vi "Remove DC Component.vi"(8 "error in":errorcluster, 10 "InverterWaveforms":T1) -> (0 "error out":errorcluster, 2 "InverterWaveforms out":T1)   [LabVIEW 2019, in "Main.lvclass"]
doc: "Developed by Kevin Thompson\nkevin@thompsonengineering.net\n\nCopyright 2020\nThompson Engineering, LLC"
uses:
  Main.lvclass
  Common/DataTypes/InverterWaveforms--cluster.ctl
  Common/DataTypes/ChannelWaveforms--cluster.ctl
  <vilib>/Analysis/NI_AALPro.lvlib
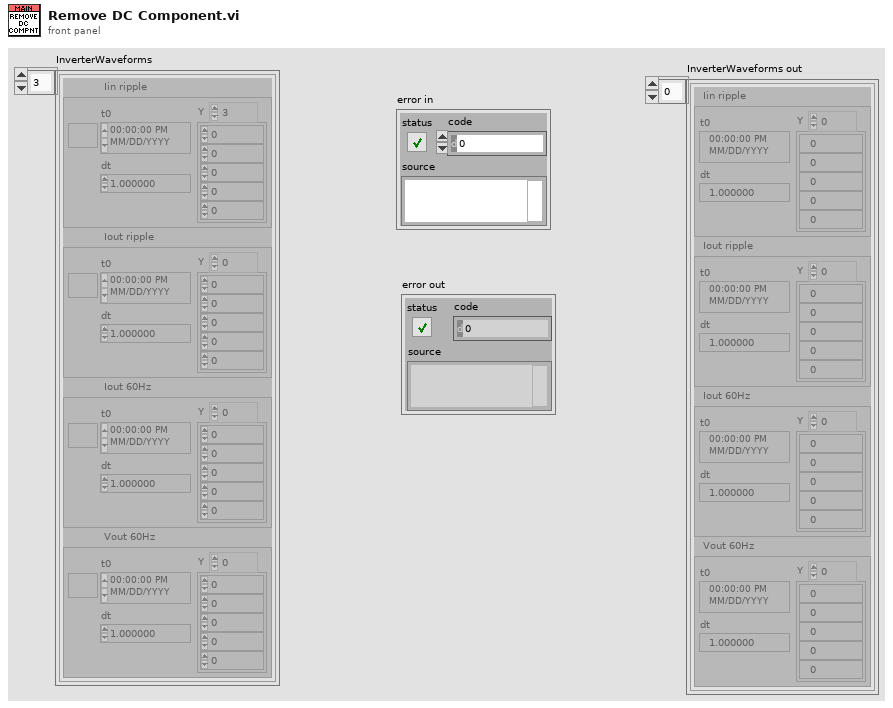
[diagram p1: front panel]
types:
  T1 = typedef "InverterWaveforms--cluster.ctl" = T2[]
  T2 = typedef "ChannelWaveforms--cluster.ctl" = cluster{"Iin ripple ":waveform(dbl), "Iout ripple ":waveform(dbl), "Iout 60Hz":waveform(dbl), "Vout 60Hz":waveform(dbl)}
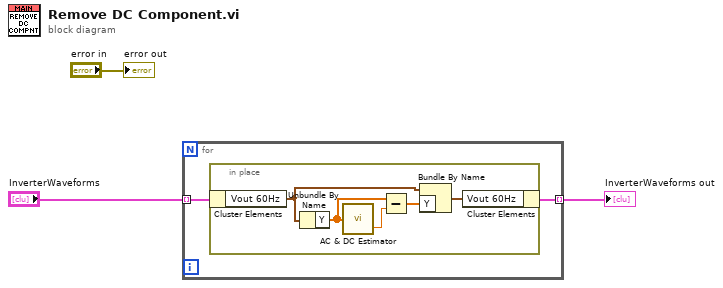
[diagram p0: block diagram]
diagram:
  n1 = for {
    tunnel: "InverterWaveforms" -> [w5] mode=indexing
    tunnel: [w4] -> w1 mode=indexing
    n2 = in-place {
      n3 = in-place-cluster #1(w5) -> ("Vout 60Hz"=w8:waveform(dbl))
      n4 = Unbundle By Name(w8) -> ("Y"=w9:dbl[])
      n5 = call <vilib>:"AC & DC Estimator.vi"("Signal (V)"=w9) -> ("DC estimate (V)"=w10:dbl)  [unwired: 1 out]
      n6 = Subtract(x=w9, y=w10) -> (x-y=w7:dbl[])
      n7 = Bundle By Name(cluster=w8, "Y"=w7) -> (w6:waveform(dbl))
      n8 = in-place-cluster #1("Vout 60Hz"=w6) -> (w4:T2)
    }
  }
  "InverterWaveforms out" <- w1
  "error out" <- "error in"
